vi "UWB communication.vi"(8 "error in (no error)":errorcluster, 11 "FPGA VI Reference In":refnum<k20>) -> (0 "error out":errorcluster, 3 "FPGA VI Reference Out":refnum<k20>)   [LabVIEW 2016]
uses:
  Typedef/UWB Cluster.ctl
  <vilib>/Utility/error.llb/Error Cluster From Error Code.vi
  <vilib>/rvi/errors/niLvFpgaAdjustHostInterfaceError.vi
  <vilib>/rvi/interface/nirviMethod/nirviMethod.xnode
  <vilib>/FPGAPlugInAG/Dynamic/niLvFpga_StartFifo_Dynamic.vi
  <vilib>/rvi/errors/niLvFpgaMergeErrorWithErrorCode.vi
  <vilib>/FPGAPlugInAG/Dynamic/niLvFpga_WriteFifo_Dynamic.vi
  <vilib>/FPGAPlugInAG/Dynamic/niLvFpga_ReadFifo_Dynamic.vi
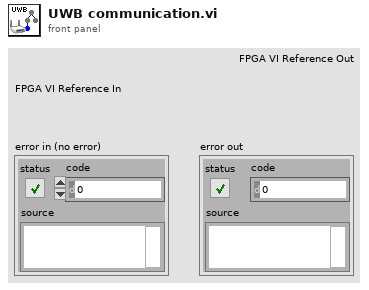
[diagram p1: front panel]
types:
  T1 = typedef "UWB Cluster.ctl" = cluster{"X":dbl, "Y":dbl, "Z":dbl, "heading":dbl, "quality":u8}
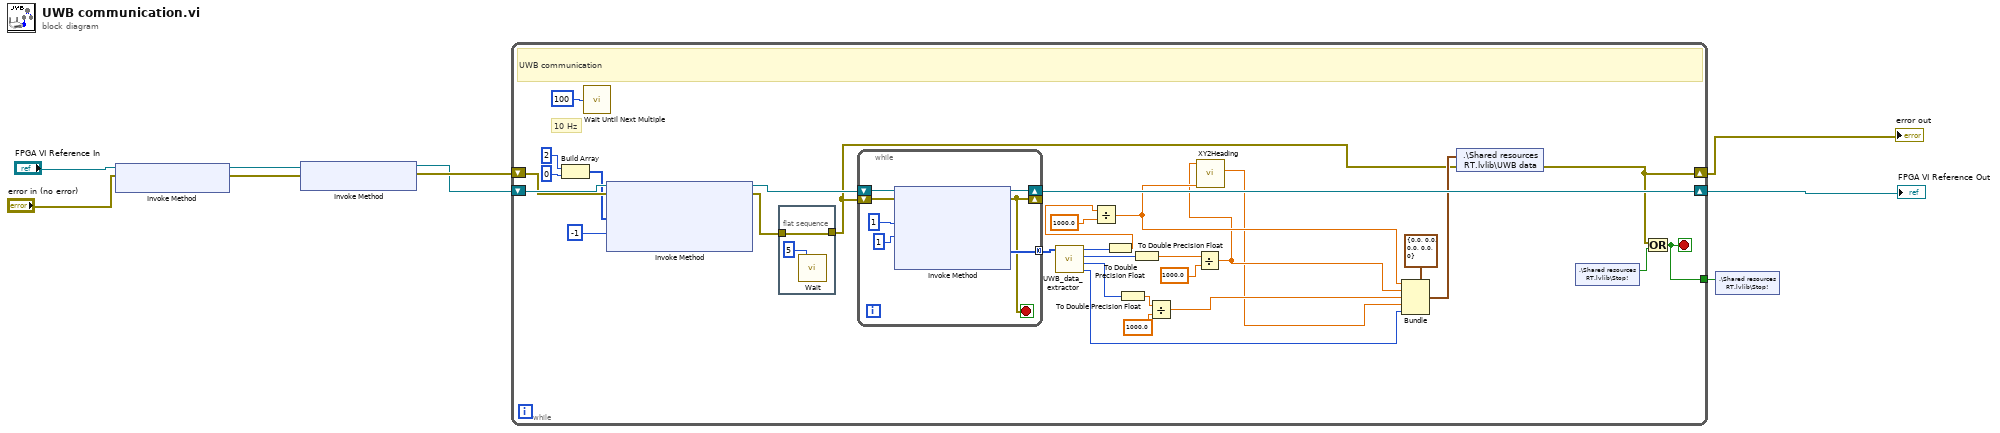
[diagram p0: block diagram]
diagram:
  n1 = xnode "Invoke Method"("FPGA VI Reference In"="FPGA VI Reference In", "error in"="error in (no error)") -> ("FPGA VI Reference Out"=w2:refnum<k20>, "error out"=w3:errorcluster)
  n2 = xnode "Invoke Method"("FPGA VI Reference In"=w2, "error in"=w3) -> ("FPGA VI Reference Out"=w4:refnum<k20>, "error out"=w5:errorcluster)
  n3 = while {
    shift-right: [w30] -> w1
    shift-left: w4 -> [w39]
    shift-right: [w12] -> w9
    shift-left: w5 -> [w35]
    tunnel: [w10] -> w8
    stop <- w10 stop-if-true
    # "10 Hz"
    # "UWB communication"
    n4 = Build Array(u8 2, u8 0) -> (w33:u8[])
    n5 = call "Wait Until Next Multiple"("Count(mSec)"=u32 100) -> ()  [unwired: 1 out]
    n6 = xnode "Invoke Method"("FPGA VI Reference In"=w39, "error in"=w35, "Data"=w33, "Timeout (ms)"=-1) -> ("FPGA VI Reference Out"=w37:refnum<k20>, "error out"=w20:errorcluster)  [unwired: 1 out]
    n7 = flat-sequence {
      tunnel: [w41] -> w13
      tunnel: w20 -> [w41]
      frame #0 {
        n8 = call "Wait"("Count(mSec)"=u32 5) -> ()  [unwired: 1 out]
      }
    }
    n9 = while {
      tunnel: [w45] -> w31 mode=concatenating
      shift-right: [w43] -> _
      shift-left: w13 -> [w49]
      shift-right: [w44] -> w30
      shift-left: w37 -> [w48]
      stop <- w43 stop-if-true
      n10 = xnode "Invoke Method"("FPGA VI Reference In"=w48, "error in"=w49, "Number of Elements"=u32 1, "Timeout (ms)"=1) -> ("FPGA VI Reference Out"=w44:refnum<k20>, "error out"=w43:errorcluster, "Data"=w45:u8[])  [unwired: 1 out]
    }
    n11 = call "UWB_data_extractor.vi"("Data"=w31) -> ("quality"=w15:u8, "Z value (mm)"=w21:i32, "Y value (mm)"=w22:i32, "X value (mm)"=w23:i32)  [unwired: 7 in]
    n12 = To Double Precision Float(number=w23) -> (double precision float=w26:dbl)
    n13 = Divide(x=w26, y=1000.0) -> (x/y=w19:dbl)
    n14 = To Double Precision Float(number=w21) -> (double precision float=w27:dbl)
    n15 = To Double Precision Float(number=w22) -> (double precision float=w25:dbl)
    n16 = Divide(x=w27, y=1000.0) -> (x/y=w17:dbl)
    n17 = Divide(x=w25, y=1000.0) -> (x/y=w18:dbl)
    n18 = call "XY2Heading.vi"("X"=w19, "Y"=w18) -> ("heading"=w16:dbl)  [unwired: 9 in]
    n19 = Bundle(cluster=T1 {"X"=0.0, "Y"=0.0, "Z"=0.0, "heading"=0.0, "quality"=0} ("UWB cluster"), "X"=w19, "Y"=w18, "Z"=w17, "heading"=w16, "quality"=w15) -> (w14:T1)
    n20 = shared-variable ".\\Shared resources RT.lvlib\\UWB data"(w14, error in=w13) -> (error out=w12:errorcluster)
    n21 = shared-variable ".\\Shared resources RT.lvlib\\Stop!"() -> (w36:bool)  [unwired: 1 in, 1 out]
    n22 = Or(x=w12, y=w36) -> (x .or. y?=w10:bool)
  }
  "error out" <- w9
  "FPGA VI Reference Out" <- w1
  n23 = shared-variable ".\\Shared resources RT.lvlib\\Stop!"(w8) -> ()  [unwired: 1 in, 1 out]
